vi "test_Write Quad Encoder Settings.vi"(8 "error in (no error)":errorcluster, 11 "TestCase in":refnum<class "FPGA Addon Speciality IO Tests.lvclass">) -> (0 "error out":errorcluster, 3 "TestCase out":refnum<class "FPGA Addon Speciality IO Tests.lvclass">)   [LabVIEW 2020, in "FPGA Addon Speciality IO Tests.lvclass"]
uses:
  FPGA Addon Speciality IO Tests.lvclass
  C:/Users/Administrator/Desktop/GIT/niveristand-custom-device-testing-tools/VeriStandTestCase/VeriStandTestCase.lvclass
  types/Channel Config.ctl
  <vilib>/addons/_JKI Toolkits/VI Tester/TestCase.llb/TestCase.lvclass
  FPGA Addon Test Class/FPGA Addon Test Class.lvclass
  C:/Program Files (x86)/National Instruments/LabVIEW 2020/vi.lib/addons/_JKI Toolkits/VI Tester/TestCase.llb/TestCase.lvclass
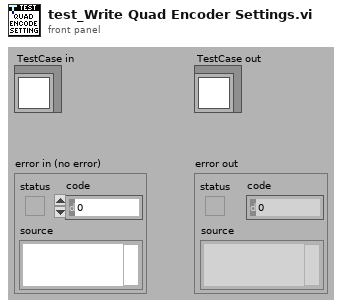
[diagram p1: front panel]
types:
  T1 = typedef "FPGA Addon Speciality IO Tests.lvclass/Channel Config.ctl" = cluster{"Scalar Output":string, "Scalar Input":string, "Value":dbl}
  T2 = typedef "NI_VS Workspace ExecutionAPI.lvlib/WorkspaceAPI.ctl" = refnum<k24>
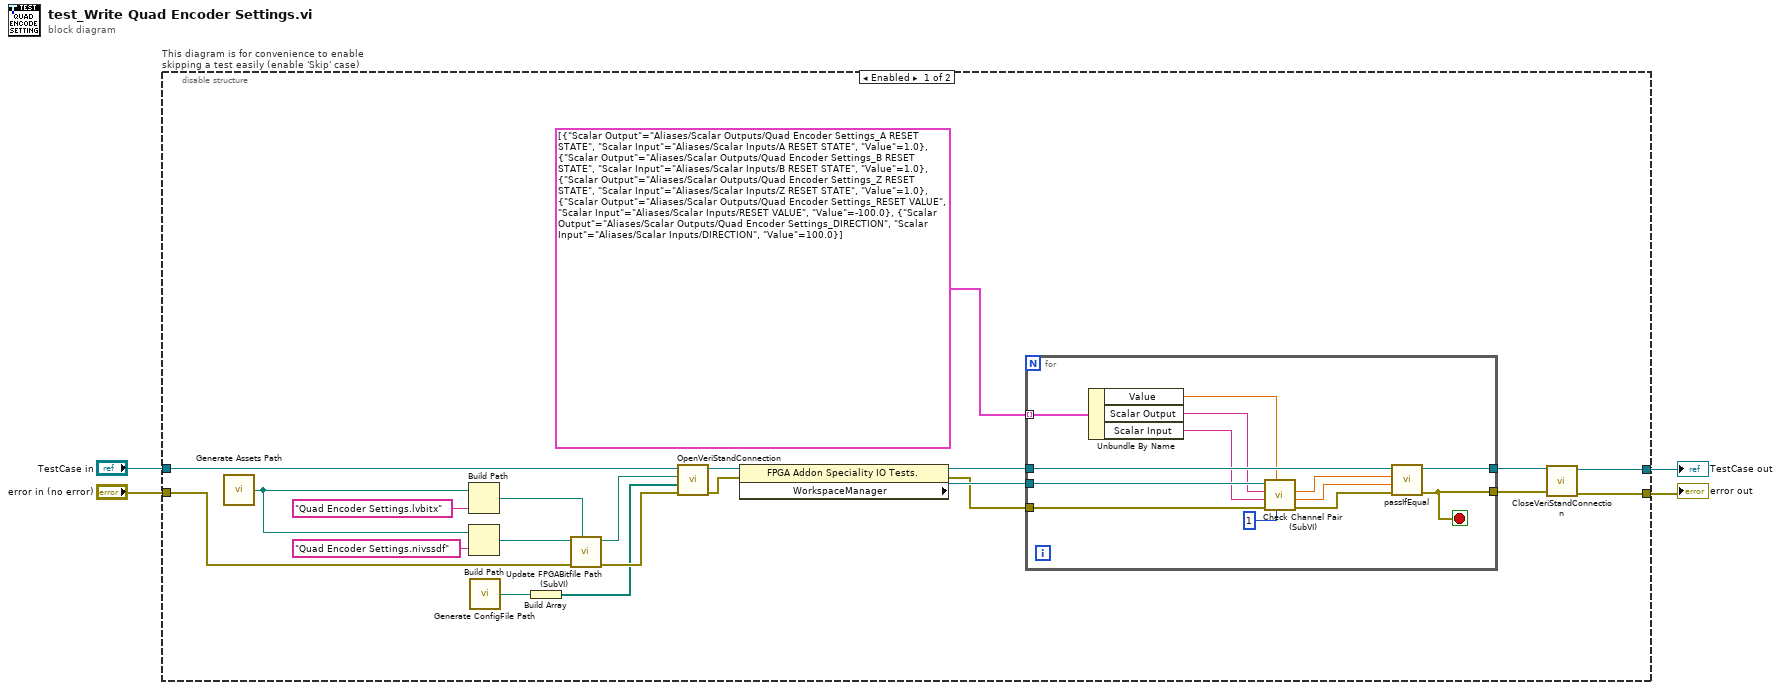
[diagram p0: block diagram]
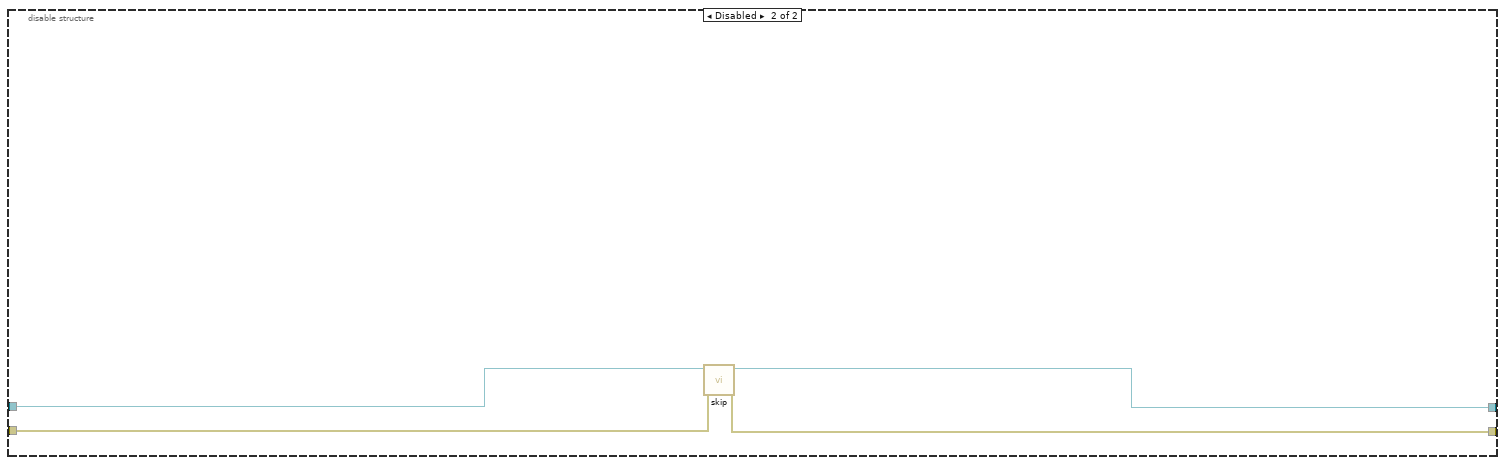
[diagram p2: hidden frame]
diagram:
  n1 = disable-structure "This diagram is for convenience to enable skipping a test easily (enable 'Skip' case)" shown="Enabled" {
    disable-tunnel: "TestCase in" -> [w20 w42]
    disable-tunnel: [w18 w40] -> w1
    disable-tunnel: [w19 w41] -> w3
    disable-tunnel: "error in (no error)" -> [w9 w39]
    frame Enabled {
      n2 = call "Generate Assets Path.vi"() -> ("Assets path"=w13:path)
      n3 = Build Path(base path=w13, name or relative path="Quad Encoder Settings.lvbitx") -> (appended path=w12:path)
      n4 = Build Path(base path=w13, name or relative path="Quad Encoder Settings.nivssdf") -> (appended path=w11:path)
      n5 = call "Generate ConfigFile Path.vi"() -> ("ConfigFile path"=w14:path)
      n6 = Build Array(w14) -> (w6:path[])
      n7 = call "Update FPGABitfile Path (SubVI).vi"("Bitfile Path"=w12, "error in (no error)"=w9, "System Definition path in"=w11) -> ("error out"=w7:errorcluster, "System Definition path out"=w5:path)  [unwired: 7 in]
      n8 = call-dynamic "OpenVeriStandConnection.vi"("error in (no error)"=w7, "overrides files"=w6, "System Definition File"=w5, "VeriStand Test Case in"=w20) -> ("error out"=w25:errorcluster, "VeriStand Test Case out"=w24:refnum<class "FPGA Addon Speciality IO Tests.lvclass">)  [unwired: 5 in, 1 out]
      n9 = property class="FPGA Addon Speciality IO Tests."(reference=w24, error in=w25) -> (reference out=w23:refnum<class "FPGA Addon Speciality IO Tests.lvclass">, error out=w21:errorcluster, "WorkspaceManager"=w22:T2)
      n10 = for {
        tunnel: w23 -> [w38]
        tunnel: w22 -> [w37]
        tunnel: w21 -> [w35]
        tunnel: T1[] [{"Scalar Output"="Aliases/Scalar Outputs/Quad Encoder Settings_A RESET STATE", "Scalar Input"="Aliases/Scalar Inputs/A RESET STATE", "Value"=1.0}, {"Scalar Output"="Aliases/Scalar Outputs/Quad Encoder Settings_B RESET STATE", "Scalar Input"="Aliases/Scalar Inputs/B RESET STATE", "Value"=1.0}, {"Scalar Output"="Aliases/Scalar Outputs/Quad Encoder Settings_Z RESET STATE", "Scalar Input"="Aliases/Scalar Inputs/Z RESET STATE", "Value"=1.0}, {"Scalar Output"="Aliases/Scalar Outputs/Quad Encoder Settings_RESET VALUE", "Scalar Input"="Aliases/Scalar Inputs/RESET VALUE", "Value"=-100.0}, {"Scalar Output"="Aliases/Scalar Outputs/Quad Encoder Settings_DIRECTION", "Scalar Input"="Aliases/Scalar Inputs/DIRECTION", "Value"=100.0}] -> [w32] mode=indexing
        tunnel: [w28] -> w16
        tunnel: [w27] -> w15
        stop <- w28 stop-if-true
        n11 = Unbundle By Name(w32) -> ("Value"=w29:dbl, "Scalar Output"=w31:string, "Scalar Input"=w30:string)
        n12 = call "Check Channel Pair (SubVI).vi"("seconds to wait"=u32 1, "OutputChannel Value in"=w29, "error in (no error)"=w35, "Input Channel"=w30, "Output Channel"=w31, "WorkspaceManager in"=w37) -> ("error out"=w36:errorcluster, "OutputChannel Value out"=w33:dbl, "InputChanel Value"=w34:dbl)  [unwired: 2 in, 1 out]
        n13 = call-dynamic "passIfEqual.vi"("error in (no error)"=w36, "y"=w33, "x"=w34, "TestCase in"=w38) -> ("error out"=w28:errorcluster, "TestCase out"=w27:refnum<class "FPGA Addon Speciality IO Tests.lvclass">)  [unwired: 6 in]
      }
      n14 = call-dynamic "CloseVeriStandConnection.vi"("error in (no error)"=w16, "VeriStand Test Case in"=w15) -> ("error out"=w19:errorcluster, "VeriStand Test Case out"=w18:refnum<class "FPGA Addon Speciality IO Tests.lvclass">)  [unwired: 8 in]
    }
    frame Disabled {
      # "skip test result while test is under development"
      n15 = call <vilib>:"skip.vi"("error in (no error)"=w39, "TestCase in"=w42) -> ("error out"=w41:errorcluster, "TestCase out"=w40:refnum<class "FPGA Addon Speciality IO Tests.lvclass">)  [unwired: 8 in]
    }
  }
  "error out" <- w3
  "TestCase out" <- w1
